vi "Set Out.vi"(8 "error in (no error)":errorcluster, 10 "Output value":refnum<class "Output Value.lvclass">, 11 "RFSoC Driver in":refnum<class "RFSoC Driver.lvclass">) -> (0 "error out":errorcluster, 3 "RFSoC Driver out":refnum<class "RFSoC Driver.lvclass">)   [LabVIEW 2019, in "RFSoC Driver.lvclass"]
uses:
  RFSoC Driver.lvclass
  Utilities/Output Value/Output Value.lvclass
  C:/GitHub/NHMFL_Core/Libraries/Instruments/Results/Acquired Result/Acquired Result.lvclass
  RFSoC Driver.lvclass/RFSoC Driver.ctl
  <vilib>/Analysis/NI_AALBase.lvlib
panel:
  out "data out":string
  out "Actual frequency":dbl format="%#_12pHz"
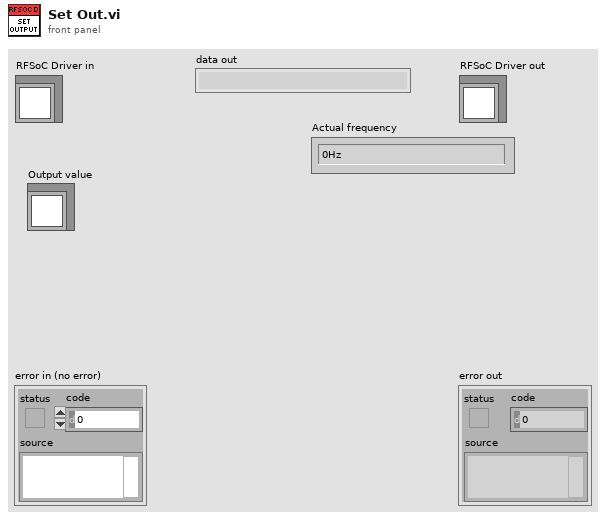
[diagram p1: front panel]
types:
  T1 = enum16{"Standard", "Buffered", "CRLF", "Immediate"}
  T2 = enum16{"big-endian, network order", "native, host order", "little-endian"}
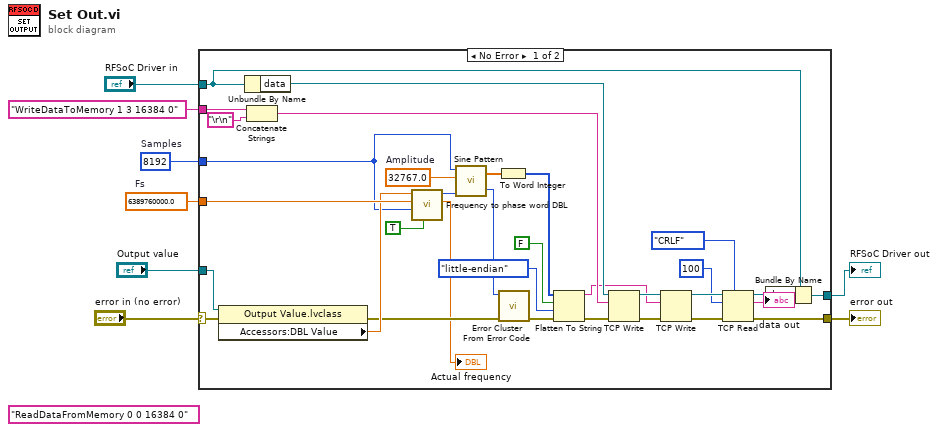
[diagram p0: block diagram]
diagram:
  (unwired) "ReadDataFromMemory 0 0 16384 0"
  w6 = 8192  # Samples
  w7 = 6389760000.0  # Fs
  n1 = case shown="No Error" "error in (no error)" {
    selector: "error in (no error)" -> [w33 w43]
    tunnel: "Output value" -> [w41 _]
    tunnel: w7 -> [w40 _]
    tunnel: w6 -> [w36 _]
    tunnel: "RFSoC Driver in" -> [w21 w42]
    tunnel: [w13 w43] -> w3
    tunnel: [w20 w42] -> w2
    tunnel: "WriteDataToMemory 1 3 16384 0" -> [w22 _]
    frame No Error {
      w35 = 32767.0  # Amplitude
      n2 = property class="Output Value.lvclass"(reference=w41, error in=w33) -> (error out=w29:errorcluster, "Accessors:DBL Value"=w39:dbl)  [unwired: 1 out]
      n3 = Unbundle By Name(w21) -> ("data"=w23:refnum<k5>)
      n4 = Concatenate Strings(w22, "\r\n") -> (w32:string)
      n5 = call "Frequency to phase word DBL.vi"("Synchonous"=TRUE, "DDS modulus"=w36, "DDS clock"=w40, "Frequency"=w39) -> ("Actual frequency"=→"Actual frequency":dbl, "Phase word"=w37:u64)  [unwired: 6 in]
      n6 = call <vilib>:"Sine Pattern.vi"("cycles"=w37, "amplitude"=w35, "samples"=w36) -> ("error"=w30:i32, "Sinusoidal Pattern"=w34:dbl[])  [unwired: 1 in]
      n7 = To Word Integer(number=w34) -> (16bit integer=w28:i16[])
      n8 = call <vilib>:"Error Cluster From Error Code.vi"("error in (no error)"=w29, "error code (0)"=w30) -> ("error out"=w26:errorcluster)  [unwired: 7 in]
      n9 = Flatten To String(anything=w28, prepend array or string size? (T)=FALSE, byte order (0:big-endian, network order)=T2."little-endian", error in (no error)=w26) -> (data string=w16:string, error out=w24:errorcluster)  [unwired: 1 out]
      n10 = TCP Write(connection ID=w23, data in=w32, error in (no error)=w24) -> (connection ID out=w17:refnum<k5>, error out=w18:errorcluster)  [unwired: 1 in, 1 out]
      n11 = TCP Write(connection ID=w17, data in=w16, error in (no error)=w18) -> (connection ID out=w15:refnum<k5>, error out=w12:errorcluster)  [unwired: 1 in, 1 out]
      n12 = TCP Read(connection ID=w15, bytes to read=100, error in (no error)=w12, 7:T1."CRLF" ("mode (standard)")) -> (connection ID out=w14:refnum<k5>, data out=→"data out":string, error out=w13:errorcluster)  [unwired: 1 in]
      n13 = Bundle By Name(cluster=w21, "data"=w14) -> (w20:refnum<class "RFSoC Driver.lvclass">)
    }
    frame Error {
    }
  }
  "error out" <- w3
  "RFSoC Driver out" <- w2
